vi "Spline Interpolant.vi"(2 "final boundary":dbl=1e+30 caption="Endgrenze" format="%0.2e", 3 "initial boundary":dbl=1e+30 caption="Anfangsgrenze" format="%0.2e", 4 "X":dbl[](array[numeric]) format="%0.2f", 5 "Y":dbl[](array[numeric]) format="%0.2f") -> (0 "error":i32 caption="Fehler", 1 "Interpolant":dbl[](array[numeric]) format="%0.2f")   [LabVIEW 2009]
doc: "Gibt ein Array <B>Interpolant</B> mit der Länge n zurück, das die zweiten Ableitungen der Spline-Interpolationsfunktion g(x) an den tabellarisierten Punkten x[i] enthält, wobei i = 0, 1,…, n 1 ist."
uses:
  C:/Program Files/National Instruments/LabVIEW 2009/resource/lvanlys.dll
panel:
  # "Spline-Interpolant"
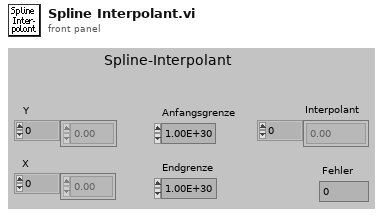
[diagram p1: front panel]
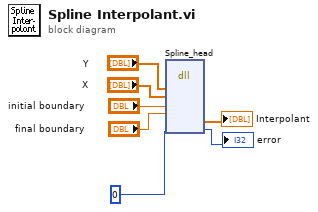
[diagram p0: block diagram]
diagram:
  n1 = dll-call lib="C:/Program Files/National Instruments/LabVIEW 2009/resource/lvanlys.*" fn="Spline_head"("Y"="Y", "X"="X", "initial boundary"="initial boundary", "final boundary"="final boundary", 0) -> ("Interpolant"=→"Interpolant":dbl[], →"error":i32)  [unwired: 9 in, 2 out]
